vi "Prototype 2.vi"() -> ()   [LabVIEW 2020]
uses:
  PI P123.01 & PiezoDrive TD250 & NI USB 7855R/PI P123.01 & PiezoDrive TD250 & NI USB 7855R.lvclass
  C:/Users/jhko7/Desktop/LabVIEW Programs/AFM Control/PZT/PZT.lvclass
  SR 830 & NI USB7855R/SR 830 & NI USB7855R.lvclass
  <vilib>/Analysis/baseanly.llb/Mean (DBL).vi
  <vilib>/addons/control/pid/pid.llb/PID (DBL).vi
  <vilib>/addons/control/pid/NI_PID_pid.lvlib
  PZT/PZT.lvclass
  <vilib>/Analysis/NI_AALBase.lvlib
panel:
  out "XY Graph":cluster{"X":dbl[], "Y":dbl[]}[](graph)
  out "standard deviation":dbl format="%0.2f"
  in  "PID gains":T1={"proportional gain (Kc)"=1.0, "integral time (Ti, min)"=0.01, "derivative time (Td, min)"=0.0} {"derivative time (Td, min)" format="%.3f"; "integral time (Ti, min)" format="%.3f"; "proportional gain (Kc)" format="%.3f"}
  in  "output range":cluster{"output high":dbl, "output low":dbl}={"output high"=100.0, "output low"=-100.0} {"output low" format="%.2f"; "output high" format="%.2f"}
  out "step size":i16
  out "error out":errorcluster
  in  "stop":bool
  out "Setpoint amplitude (V)":dbl
  in  "error in":errorcluster
  out "Amplitude (V rms)":dbl
  out "Z voltage (bits)":i16
  in  "setpoint ratio (%)":dbl
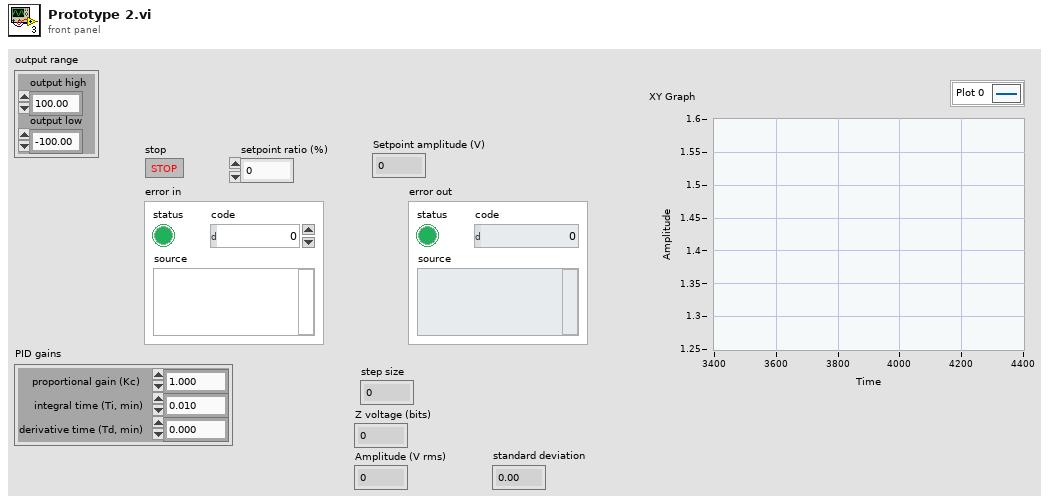
[diagram p1: front panel]
types:
  T1 = cluster{"proportional gain (Kc)":dbl, "integral time (Ti, min)":dbl, "derivative time (Td, min)":dbl}
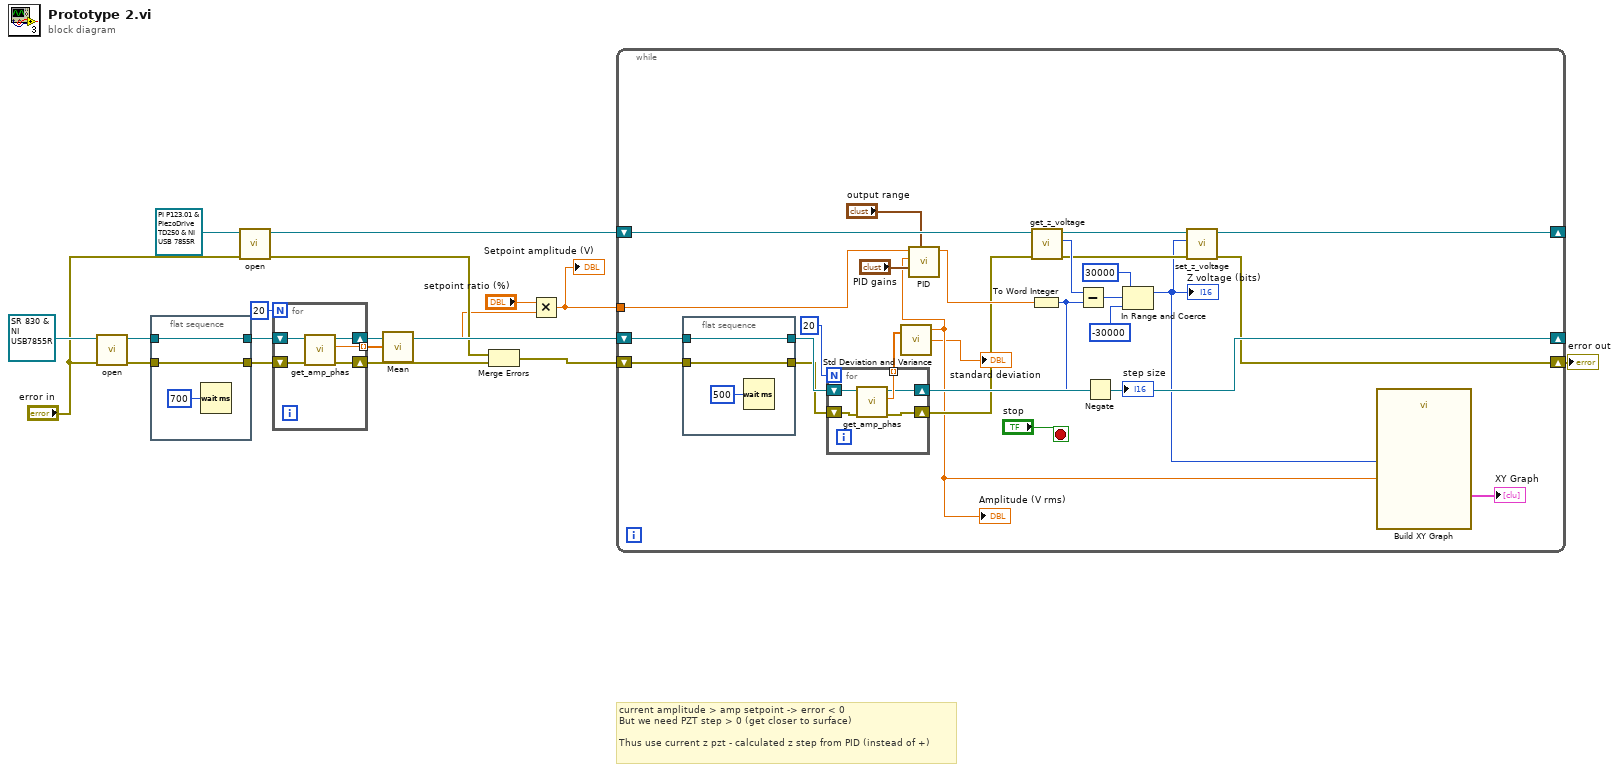
[diagram p0: block diagram]
diagram:
  # "current amplitude > amp setpoint -> error < 0\nBut we need PZT step > 0 (get closer to surface)\n\nThus use current z pzt - calculated z step from PID (instead of +)"
  n1 = call-dynamic "open.vi"("error in (no error)"="error in", "Instrument in"=refnum<class "SR 830 & NI USB7855R.lvclass"> refnum ("SR 830 & NI USB7855R.lvclass")) -> ("error out"=w5:errorcluster, "Instrument out"=w7:refnum<class "SR 830 & NI USB7855R.lvclass">)  [unwired: 8 in]
  n2 = flat-sequence {
    tunnel: w7 -> [w21]
    tunnel: [w21] -> w6
    tunnel: w5 -> [w20]
    tunnel: [w20] -> w4
    frame #0 {
      n3 = Wait (ms)(milliseconds to wait=u32 700) -> ()  [unwired: 1 out]
    }
  }
  n4 = call-dynamic "open.vi"("error in (no error)"="error in", "PI P123.01 & PiezoDrive TD250 & NI USB 7855R in"=refnum<class "PI P123.01 & PiezoDrive TD250 & NI USB 7855R.lvclass"> refnum ("PI P123.01 & PiezoDrive TD250 & NI USB 7855R.lvclass")) -> ("error out"=w11:errorcluster, "PI P123.01 & PiezoDrive TD250 & NI USB 7855R out"=w13:refnum<class "PI P123.01 & PiezoDrive TD250 & NI USB 7855R.lvclass">)  [unwired: 8 in]
  n5 = for {
    N: 20 -> [_]
    tunnel: [w26] -> w3 mode=indexing
    shift-right: [w25] -> w17
    shift-left: w6 -> [w23]
    shift-right: [w24] -> w10
    shift-left: w4 -> [w22]
    n6 = call-dynamic "get_amp_phas.vi"("error in (no error)"=w22, "SR 830 & NI USB7855R in"=w23) -> ("error out"=w24:errorcluster, "Amplitude (V rms)"=w26:dbl, "SR 830 & NI USB7855R out"=w25:refnum<class "SR 830 & NI USB7855R.lvclass">)  [unwired: 6 in, 1 out]
  }
  n7 = call-poly <vilib>:"Mean.vi"("X"=w3) -> ("mean"=w2:dbl)  [unwired: 1 out]
  n8 = Merge Errors(w11, w10) -> (w9:errorcluster)
  n9 = Multiply(x="setpoint ratio (%)", y=w2) -> (x*y=w12:dbl)
  "Setpoint amplitude (V)" <- w12
  n10 = while {
    tunnel: w12 -> [w54]
    shift-right: [w51] -> _
    shift-left: w17 -> [w39]
    shift-right: [w48] -> _
    shift-left: w13 -> [w50]
    shift-right: [w45] -> w8
    shift-left: w9 -> [w38]
    stop <- "stop" stop-if-true
    n11 = flat-sequence {
      tunnel: w39 -> [w62]
      tunnel: w38 -> [w61]
      tunnel: [w62] -> w37
      tunnel: [w61] -> w36
      frame #0 {
        n12 = Wait (ms)(milliseconds to wait=u32 500) -> ()  [unwired: 1 out]
      }
    }
    n13 = for {
      N: 20 -> [_]
      tunnel: [w59] -> w30 mode=indexing
      shift-right: [w58] -> w51
      shift-left: w37 -> [w56]
      shift-right: [w57] -> w47
      shift-left: w36 -> [w55]
      n14 = call-dynamic "get_amp_phas.vi"("error in (no error)"=w55, "SR 830 & NI USB7855R in"=w56) -> ("error out"=w57:errorcluster, "Amplitude (V rms)"=w59:dbl, "SR 830 & NI USB7855R out"=w58:refnum<class "SR 830 & NI USB7855R.lvclass">)  [unwired: 6 in, 1 out]
    }
    n15 = call <vilib>:"Std Deviation and Variance.vi"("X"=w30) -> ("mean"=w29:dbl, "standard deviation"=→"standard deviation":dbl)  [unwired: 1 in, 1 out]
    "Amplitude (V rms)" <- w29
    n16 = call-poly <vilib>:"PID.vi"("output range"="output range", "PID gains"="PID gains", "process variable"=w29, "setpoint"=w54) -> ("output"=w53:dbl)  [unwired: 6 in, 1 out]
    n17 = To Word Integer(number=w53) -> (16bit integer=w42:i16)
    n18 = call "get_z_voltage.vi"("error in"=w47, "PZT in"=w50) -> ("error out"=w46:errorcluster, "Z Voltage out"=w52:i16, "PZT out"=w49:refnum<class "PI P123.01 & PiezoDrive TD250 & NI USB 7855R.lvclass">)  [unwired: 7 in]
    n19 = Subtract(x=w52, y=w42) -> (x-y=w35:i16)
    n20 = Negate(x=w42) -> (-x=→"step size":i16)
    n21 = In Range and Coerce(upper limit=i16 30000, x=w35, lower limit=i16 -30000) -> (coerced(x)=w32:i16)  [unwired: 1 out]
    "Z voltage (bits)" <- w32
    n22 = call-dynamic "set_z_voltage.vi"("error in (no error)"=w46, "Z voltage (bits)"=w32, "PI P123.01 & PiezoDrive TD250 & NI USB 7855R in"=w49) -> ("error out"=w45:errorcluster, "PI P123.01 & PiezoDrive TD250 & NI USB 7855R out"=w48:refnum<class "PI P123.01 & PiezoDrive TD250 & NI USB 7855R.lvclass">)  [unwired: 7 in]
    n23 = call "Build XY Graph"("Y Input"=w29, "X Input"=w32) -> ("XY Graph"=→"XY Graph":cluster{"X":dbl[], "Y":dbl[]}[])  [unwired: 8 in, 1 out]
  }
  "error out" <- w8
